vi "Cases.vi"() -> ()   [LabVIEW 2020]
panel:
  out "Resultadeishon 2":dbl format="%#_13g"
  in  "Valor 5":dbl format="%#_13g"
  in  "Valor 4":dbl format="%#_13g"
  in  "Enum":enum16{"Multi", "Resta", "Add"}(ring)
  out "Resultadeishon":dbl format="%#_13g"
  in  "Valor 3":dbl format="%#_13g"
  in  "Valor 3":dbl format="%#_13g"
  in  "Case selector":string
  out "Resultado":dbl
  in  "Valor 2":dbl format="%#_13g"
  in  "Valor 1":dbl format="%#_13g"
  in  "Case selector":i32
  in  "Case con cluster de error":errorcluster
  out "Numeric":dbl
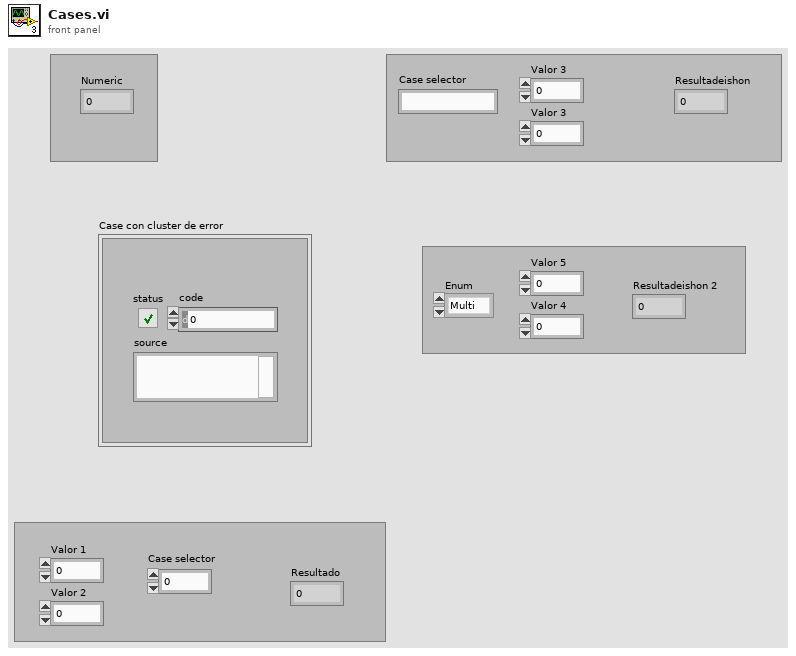
[diagram p1: front panel]
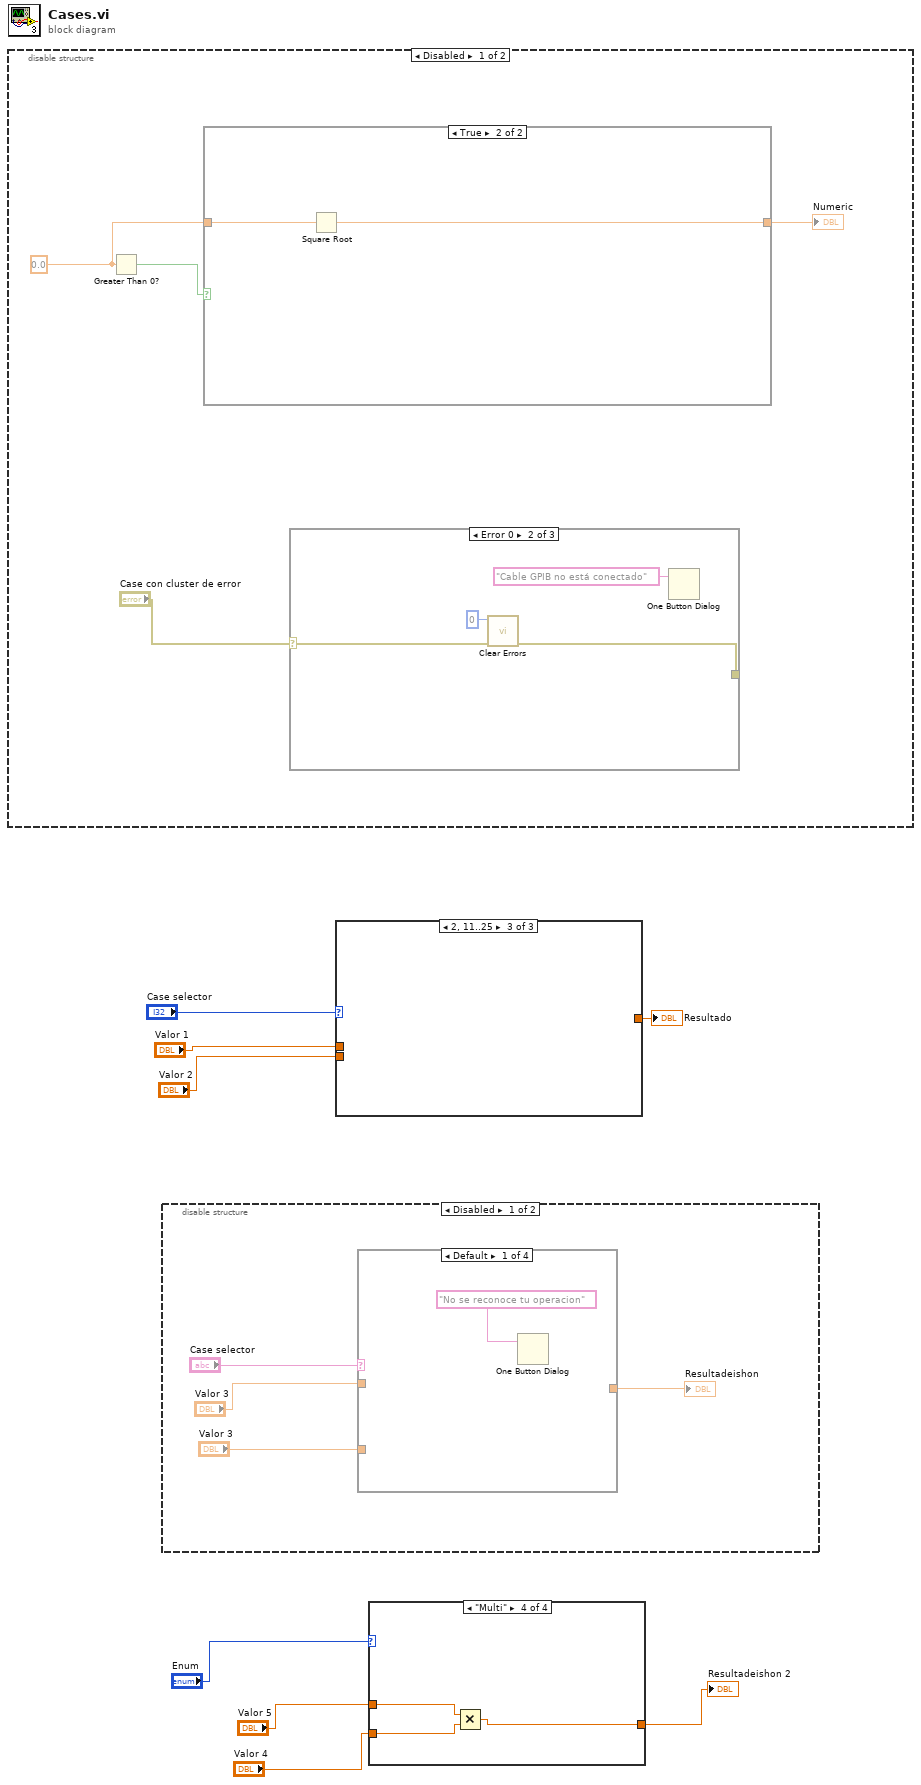
[diagram p0: block diagram]
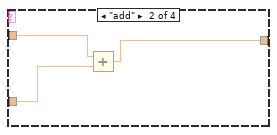
[diagram p2: hidden frame]
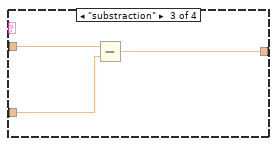
[diagram p3: hidden frame]
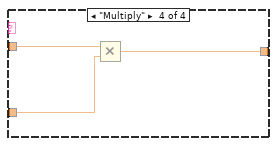
[diagram p4: hidden frame]
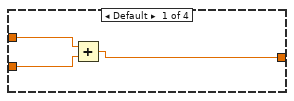
[diagram p6: hidden frame]
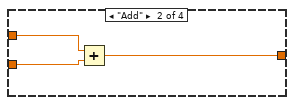
[diagram p7: hidden frame]
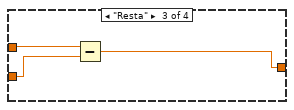
[diagram p8: hidden frame]
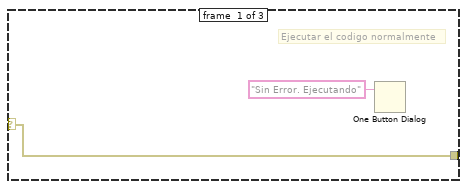
[diagram p9: hidden frame]
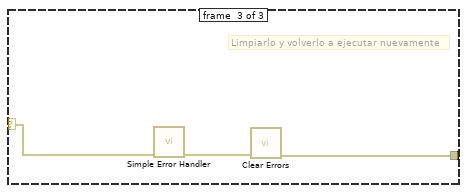
[diagram p10: hidden frame]
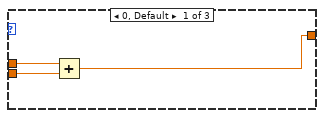
[diagram p13: hidden frame]
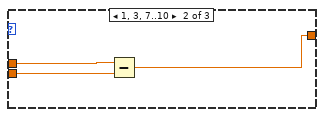
[diagram p14: hidden frame]
diagram:
  n1 = disable-structure shown="Disabled" {
    frame Disabled {
      w12 = 0.0
      n2 = Greater Than 0?(x=w12) -> (x > 0?=w10:bool)
      n3 = case shown="True" w10 {
        tunnel: w12 -> [_ w23]
        tunnel: [_ w22] -> w11
        frame False {
        }
        frame True {
          n4 = Square Root(x=w23) -> (sqrt(x)=w22:dbl)
        }
      }
      "Numeric" <- w11
      n5 = case shown="Error 0" "Case con cluster de error" {
        selector: "Case con cluster de error" -> [w13 w18 w21]
        tunnel: [w13 w17 w19] -> _
        frame #0 {
          # "Ejecutar el codigo normalmente"
          n6 = One Button Dialog(message="Sin Error. Ejecutando") -> ()  [unwired: 1 in, 1 out]
        }
        frame #1 {
          n7 = call <vilib>:"Clear Errors.vi"("error in (no error)"=w18, "specific error code to clear (0: all)"=0) -> ("error out"=w17:errorcluster)  [unwired: 4 in, 1 out]
          n8 = One Button Dialog(message="Cable GPIB no está conectado") -> ()  [unwired: 1 in, 1 out]
        }
        frame #2 {
          # "Limpiarlo y volverlo a ejecutar nuevamente"
          n9 = call <vilib>:"Simple Error Handler.vi"("error in (no error)"=w21) -> ("error out"=w20:errorcluster)  [unwired: 4 in, 4 out]
          n10 = call <vilib>:"Clear Errors.vi"("error in (no error)"=w20) -> ("error out"=w19:errorcluster)  [unwired: 5 in, 1 out]
        }
      }
    }
    frame Enabled {
    }
  }
  n11 = disable-structure shown="Disabled" {
    frame Disabled {
      n12 = case shown="Default" "Case selector" {
        tunnel: "Valor 3" -> [_ w31 w34 w37]
        tunnel: "Valor 3" -> [_ w30 w33 w36]
        tunnel: [_ w29 w32 w35] -> w24
        frame Default {
          n13 = One Button Dialog(message="No se reconoce tu operacion") -> ()  [unwired: 1 in, 1 out]
        }
        frame "add" {
          n14 = Add(x=w31, y=w30) -> (x+y=w29:dbl)
        }
        frame "substraction" {
          n15 = Subtract(x=w34, y=w33) -> (x-y=w32:dbl)
        }
        frame "Multiply" {
          n16 = Multiply(x=w37, y=w36) -> (x*y=w35:dbl)
        }
      }
      "Resultadeishon" <- w24
    }
    frame Enabled {
    }
  }
  n17 = case shown="2, 11..25" "Case selector" {
    tunnel: "Valor 1" -> [w40 w43 _]
    tunnel: "Valor 2" -> [w39 w42 _]
    tunnel: [w38 w41 _] -> w5
    frame 0, Default {
      n18 = Add(x=w40, y=w39) -> (x+y=w38:dbl)
    }
    frame 1, 3, 7..10 {
      n19 = Subtract(x=w43, y=w42) -> (x-y=w41:dbl)
    }
    frame 2, 11..25 {
    }
  }
  "Resultado" <- w5
  n20 = case shown="\"Multi\"" "Enum" {
    tunnel: "Valor 5" -> [w45 w49 w51 w54]
    tunnel: "Valor 4" -> [w46 w48 w52 w55]
    tunnel: [w44 w47 w50 w53] -> w1
    frame Default {
      n21 = Add(x=w45, y=w46) -> (x+y=w44:dbl)
    }
    frame "Add" {
      n22 = Add(x=w49, y=w48) -> (x+y=w47:dbl)
    }
    frame "Resta" {
      n23 = Subtract(x=w51, y=w52) -> (x-y=w50:dbl)
    }
    frame "Multi" {
      n24 = Multiply(x=w54, y=w55) -> (x*y=w53:dbl)
    }
  }
  "Resultadeishon 2" <- w1
